vi "Write UserInterfaceDetails.vi"(8 "error in (no error)":errorcluster, 10 "ni_measurements_v1_UserInterfaceDetails":T1, 11 "MeasurementService in":refnum<class "MeasurementService.lvclass">) -> (0 "error out":errorcluster, 3 "MeasurementService out":refnum<class "MeasurementService.lvclass">)   [LabVIEW 2020, in "Load Regulation.lvlib" / "MeasurementService.lvclass"]
uses:
  MeasurementService.lvclass
  RPC Messages/ni_measurements_v1_UserInterfaceDetails.ctl
  MeasurementService.lvclass/MeasurementService.ctl
  Load Regulation.lvlib
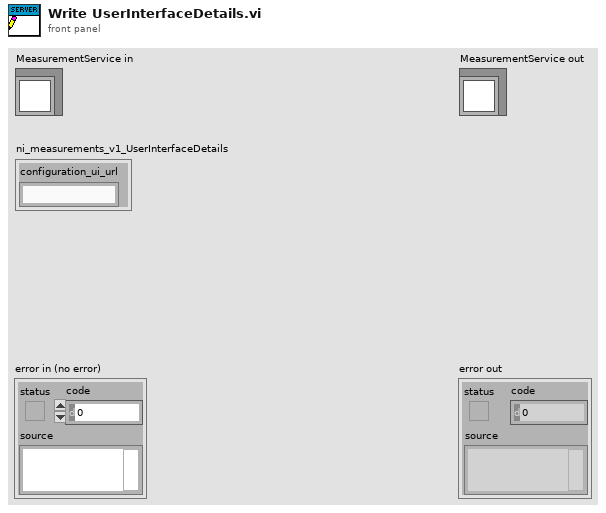
[diagram p1: front panel]
types:
  T1 = typedef "Load Regulation.lvlib/ni_measurements_v1_UserInterfaceDetails.ctl" = cluster{"configuration_ui_url":string}
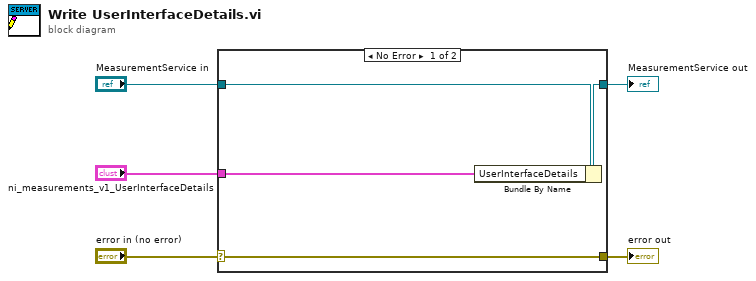
[diagram p0: block diagram]
diagram:
  n1 = case shown="No Error" "error in (no error)" {
    selector: "error in (no error)" -> [w9 w10]
    tunnel: [w9 w10] -> w4
    tunnel: [w7 w11] -> w2
    tunnel: "MeasurementService in" -> [w8 w11]
    tunnel: "ni_measurements_v1_UserInterfaceDetails" -> [w6 _]
    frame No Error {
      n2 = Bundle By Name(cluster=w8, "UserInterfaceDetails"=w6) -> (w7:refnum<class "MeasurementService.lvclass">)
    }
    frame Error {
    }
  }
  "error out" <- w4
  "MeasurementService out" <- w2
